vi "Voc (SubVI) RT.vi"(1 "Actual SOC( / )":dbl) -> (0 "Voc":dbl)   [LabVIEW 2017]
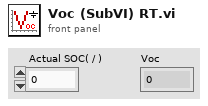
[diagram p1: front panel]
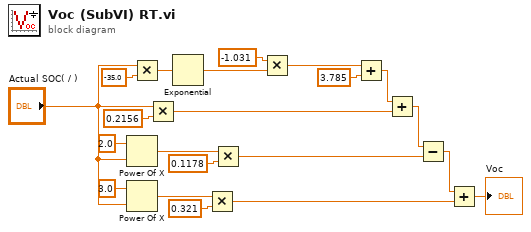
[diagram p0: block diagram]
diagram:
  n1 = Power Of X(1:"Actual SOC( / )", 2:2.0 ("y")) -> (0:w8:dbl)
  n2 = Power Of X(1:"Actual SOC( / )", 2:3.0 ("y")) -> (0:w3:dbl)
  n3 = Multiply(x="Actual SOC( / )", y=-35.0) -> (x*y=w18:dbl)
  n4 = Multiply(x="Actual SOC( / )", y=0.2156) -> (x*y=w12:dbl)
  n5 = Exponential(1:w18) -> (0:w16:dbl)
  n6 = Multiply(x=w3, y=0.321) -> (x*y=w2:dbl)
  n7 = Multiply(x=w8, y=0.1178) -> (x*y=w7:dbl)
  n8 = Multiply(x=-1.031, y=w16) -> (x*y=w14:dbl)
  n9 = Add(x=w14, y=3.785) -> (x+y=w11:dbl)
  n10 = Add(x=w11, y=w12) -> (x+y=w6:dbl)
  n11 = Subtract(x=w6, y=w7) -> (x-y=w1:dbl)
  n12 = Add(x=w1, y=w2) -> (x+y=→"Voc":dbl)
